vi "Write Startup INI.vi"(8 "error in (no error)":errorcluster, 10 "Startup INI":T1={"ConfigFolder"=path "C:/Projects/BRS_V3/Configuration", "DataFolder"=path "C:/Projects/BRS_V3/Data", "LogFolder"=path "C:/Projects/BRS_V3/Log", "DocFolder"=path "C:/Projects/BRS_V3/Documents", "AutomationFolder"=path "C:/Projects/BRS_V3/Automation", "SubsystemPathList"=[path "C:/Projects/BRS_V3/Source/Subsystems", path "C:/Projects/BRS_V3/Source/Core", path "C:/Projects/Seminet_Common/Subsystem"], "SystemStartup"="", "MainUI"="", "SystemConfigFJilename"="BRS_V3.xml", "IOConfigFileFilename"="IOConfig.xml", "SystemSimulation"=FALSE}, 11 "Startup INI file":path=path "C:/Projects/BRS_V3/startup.ini") -> (0 "error out":errorcluster)   [LabVIEW 2020]
doc: "Developed by Kevin Thompson\nkevin@thompsonengineering.net\n\nCopyright 2018-2020\nThompson Engineering, LLC"
uses:
  DataTypes/Startup INI Data--cluster.ctl
  <vilib>/Utility/config.llb/NI_LVConfig.lvlib
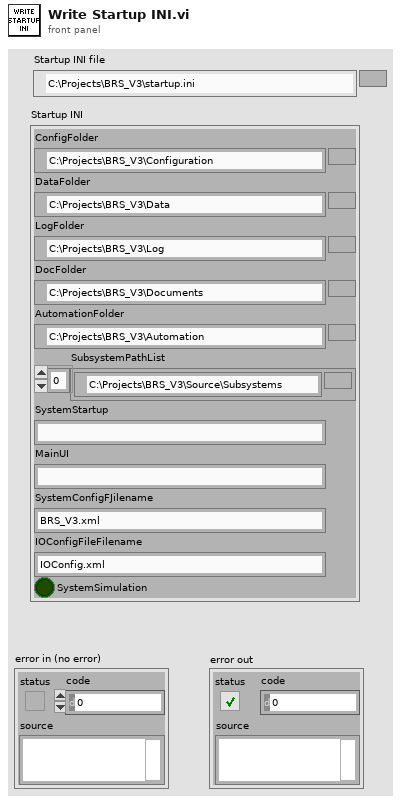
[diagram p1: front panel]
types:
  T1 = typedef "Startup INI Data--cluster.ctl" = cluster{"ConfigFolder":path, "DataFolder":path, "LogFolder":path, "DocFolder":path, "AutomationFolder":path, "SubsystemPathList":path[], "SystemStartup":string, "MainUI":string, "SystemConfigFJilename":string, "IOConfigFileFilename":string, "SystemSimulation":bool}
  T2 = typedef "NI_LVConfig.lvlib/Config Data RefNum.ctl" = refnum<k1>
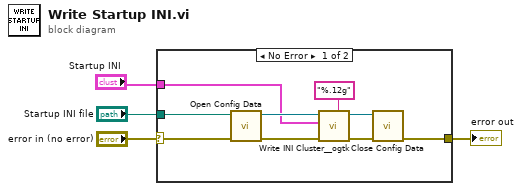
[diagram p0: block diagram]
diagram:
  n1 = case shown="No Error" "error in (no error)" {
    selector: "error in (no error)" -> [w7 w14]
    tunnel: "Startup INI" -> [w8 _]
    tunnel: [w6 w14] -> w2
    tunnel: "Startup INI file" -> [w5 _]
    frame No Error {
      n2 = call <vilib>:"Open Config Data.vi"("error in (no error)"=w7, "configuration file path"=w5) -> ("error out"=w12:errorcluster, "refnum"=w11:T2)  [unwired: 7 in, 1 out]
      n3 = call <userlib>:"Write INI Cluster__ogtk.vi"("float number format (optional)"="%.12g", "error in (no error)"=w12, "INI Fomatted Cluster"=w8, "refnum"=w11) -> ("error out"=w10:errorcluster, "dup refnum"=w9:T2)  [unwired: 6 in]
      n4 = call <vilib>:"Close Config Data.vi"("error in (no error)"=w10, "refnum"=w9) -> ("error out"=w6:errorcluster)  [unwired: 8 in, 1 out]
    }
    frame Error {
    }
  }
  "error out" <- w2
